vi "sensor cmd time set.vi"(4 "second":u32, 5 "minute":u32, 6 "hour":u32, 7 "day":u32, 9 "month":u32, 10 "year":u32, 11 "device_handle":u32) -> (2 "function return":i32, 3 "device_handle out":u32)   [LabVIEW 2019, in "apdm.lvlib"]
doc: "APDM_EXPORT int apdm_sensor_cmd_time_set(apdm_device_handle_t device_handle, uint32_t year, uint32_t month, uint32_t day, uint32_t hour, uint32_t minute, uint32_t second);"
uses:
  apdm.lvlib
  Lee Lab/CP FES Walking 2018/Code/Working/LabVIEW/apdm.dll
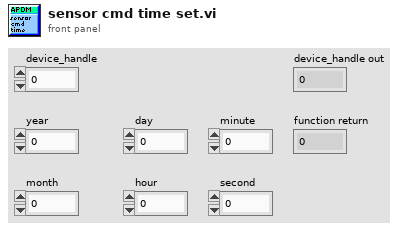
[diagram p1: front panel]
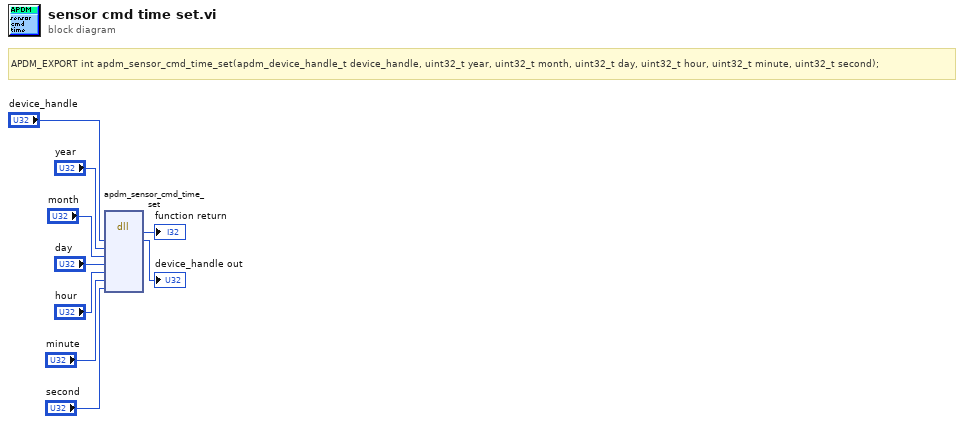
[diagram p0: block diagram]
diagram:
  # "APDM_EXPORT int apdm_sensor_cmd_time_set(apdm_device_handle_t device_handle, uint32_t year, uint32_t month, uint32_t day, uint32_t hour, uint32_t minute, uint32_t second);"
  n1 = dll-call lib="C:/Users/jfalesi/Dropbox/Lee Lab/CP FES Walking 2018/Code/Working/LabVIEW/apdm.*" fn="apdm_sensor_cmd_time_set"("device_handle"="device_handle", "year"="year", "month"="month", "day"="day", "hour"="hour", "minute"="minute", "second"="second") -> (→"function return":i32, "device_handle"=→"device_handle out":u32)  [unwired: 9 in, 2 out]
